vi "FTW-Ether-Configuration-Populate.vi"(5 "Configuration String":string, 11 "error in":errorcluster) -> (6 "Filled Configuration String":string, 15 "error out":errorcluster)   [LabVIEW 2013, in "FTW-Ether.lvclass"]
uses:
  FTW-Ether.lvclass
  JSON/FTW-JSON-UpdateMode.ctl
  JSON/FTW-JSON.lvclass
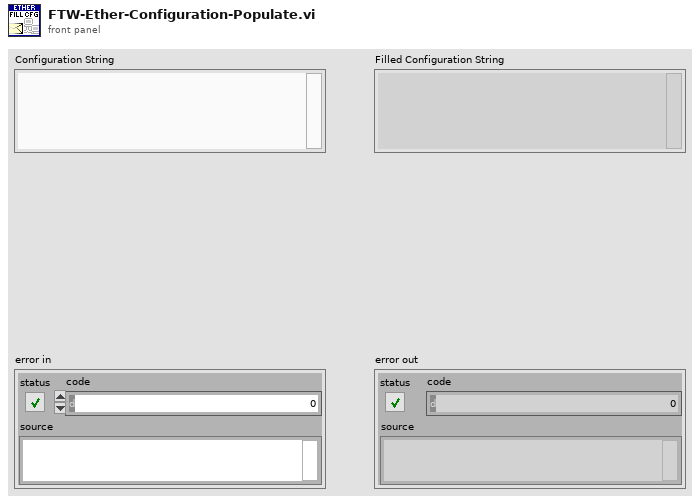
[diagram p1: front panel]
types:
  T1 = typedef "FTW-JSON.lvclass/FTW-JSON-UpdateMode.ctl" = enum16{"Upsert", "Update Only", "Insert Only"}
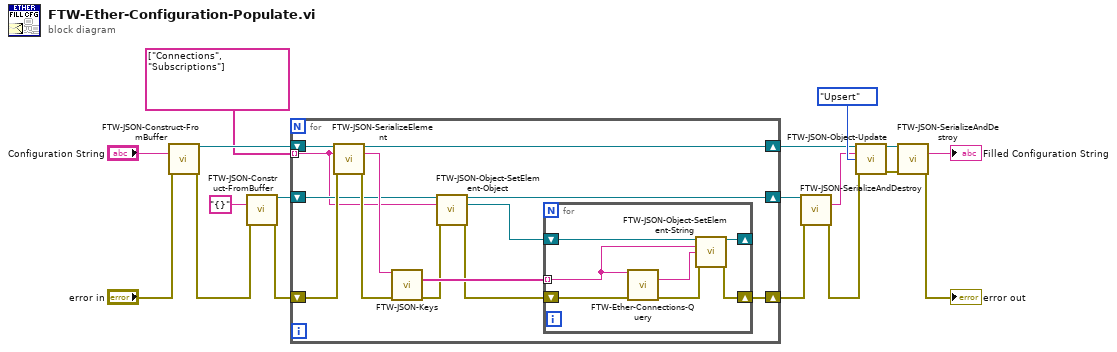
[diagram p0: block diagram]
diagram:
  n1 = call "FTW-JSON-Construct-FromBuffer.vi"("JSON String (UTF-8)"="Configuration String", "error in"="error in") -> ("JSON Object"=w16:refnum<class "FTW-JSON.lvclass">, "error out"=w7:errorcluster)  [unwired: 12 in]
  n2 = call "FTW-JSON-Construct-FromBuffer.vi"("JSON String (UTF-8)"="{}", "error in"=w7) -> ("JSON Object"=w15:refnum<class "FTW-JSON.lvclass">, "error out"=w6:errorcluster)  [unwired: 12 in]
  n3 = for {
    tunnel: string[] ["Connections", "Subscriptions"] -> [w21] mode=indexing
    shift-right: [w19] -> w5
    shift-left: w15 -> [w22]
    shift-right: [w24] -> w4
    shift-left: w6 -> [w31]
    shift-right: [w25] -> w14
    shift-left: w16 -> [w29]
    n4 = call "FTW-JSON-SerializeElement.vi"("JSON Object"=w29, "Key"=w21, "error in"=w31) -> ("JSON Object"=w25:refnum<class "FTW-JSON.lvclass">, "Element as JSON String"=w28:string, "error out"=w30:errorcluster)  [unwired: 9 in, 1 out]
    n5 = call "FTW-JSON-Keys.vi"("JSON Opject"=w28, "error in"=w30) -> ("Keys"=w27:string[], "error out"=w26:errorcluster)  [unwired: 11 in, 1 out]
    n6 = call "FTW-JSON-Object-SetElement-Object.vi"("JSON Object"=w22, "Key"=w21, "error in"=w26) -> ("JSON Root Object"=w19:refnum<class "FTW-JSON.lvclass">, "JSON Sub-Object"=w20:refnum<class "FTW-JSON.lvclass">, "error out"=w23:errorcluster)  [unwired: 10 in]
    n7 = for {
      tunnel: w27 -> [w33] mode=indexing
      shift-right: [w38] -> _
      shift-left: w20 -> [w35]
      shift-right: [w36] -> w24
      shift-left: w23 -> [w37]
      n8 = call "FTW-Ether-Connections-Query.vi"("Connection"=w33, "error in"=w37) -> ("Fetched Address"=w32:string, "error out"=w34:errorcluster)  [unwired: 12 in]
      n9 = call "FTW-JSON-Object-SetElement-String.vi"("JSON Object"=w35, "Key"=w33, "Value"=w32, "error in"=w34) -> ("JSON Object out"=w38:refnum<class "FTW-JSON.lvclass">, "error out"=w36:errorcluster)  [unwired: 10 in]
    }
  }
  n10 = call "FTW-JSON-SerializeAndDestroy.vi"("JSON Object"=w5, "error in"=w4) -> ("JSON String (UTF-8)"=w2:string, "error out"=w3:errorcluster)  [unwired: 12 in]
  n11 = call "FTW-JSON-Object-Update.vi"("JSON Object"=w14, "JSON Object to Merge"=w2, "Update Mode"=FTW-JSON-UpdateMode."Upsert", "error in"=w3) -> ("JSON Object out"=w12:refnum<class "FTW-JSON.lvclass">, "error out"=w13:errorcluster)  [unwired: 10 in]
  n12 = call "FTW-JSON-SerializeAndDestroy.vi"("JSON Object"=w12, "error in"=w13) -> ("JSON String (UTF-8)"=→"Filled Configuration String":string, "error out"=→"error out":errorcluster)  [unwired: 12 in]
